vi "AuMT8852B SCO Input Sample Size.vi"(5 "Size (8-bit)":enum16{"8-bit", "16-bit"}(ring), 7 "Set/Get (Set)":enum16{"Set", "Get"}(ring), 8 "error in (no error)":errorcluster, 11 "VISA session":refnum<visa-resource-name>) -> (0 "error out":errorcluster, 2 "error code":i32, 3 "VISA session out":refnum<visa-resource-name>, 4 "Size out":enum16{"8-bit", "16-bit"}(ring))   [LabVIEW 2017]
doc: "Anritsu MT8852B Bluetooth Tester\n\nThis command is used to set the input sample size for the audio connection to either 8 bit or 16 bit. The value is only used by the MT885x when it is controlling an EUT via the front panel connection. The command can only be used when there is an ACL connection (and if the EUT is controlled via the front panel, no SCO connection).\n\nINPUTS\nSet/Get - whether the value is being sent to or retrieved from the instrument.\nSize - information to send to the instrument.\n\nOUTPUTS\nSize out - the present value in the instrument."
uses:
  <instrlib>/aumt8852B/General/Utilities/MT8850 Attribute ID.ctl
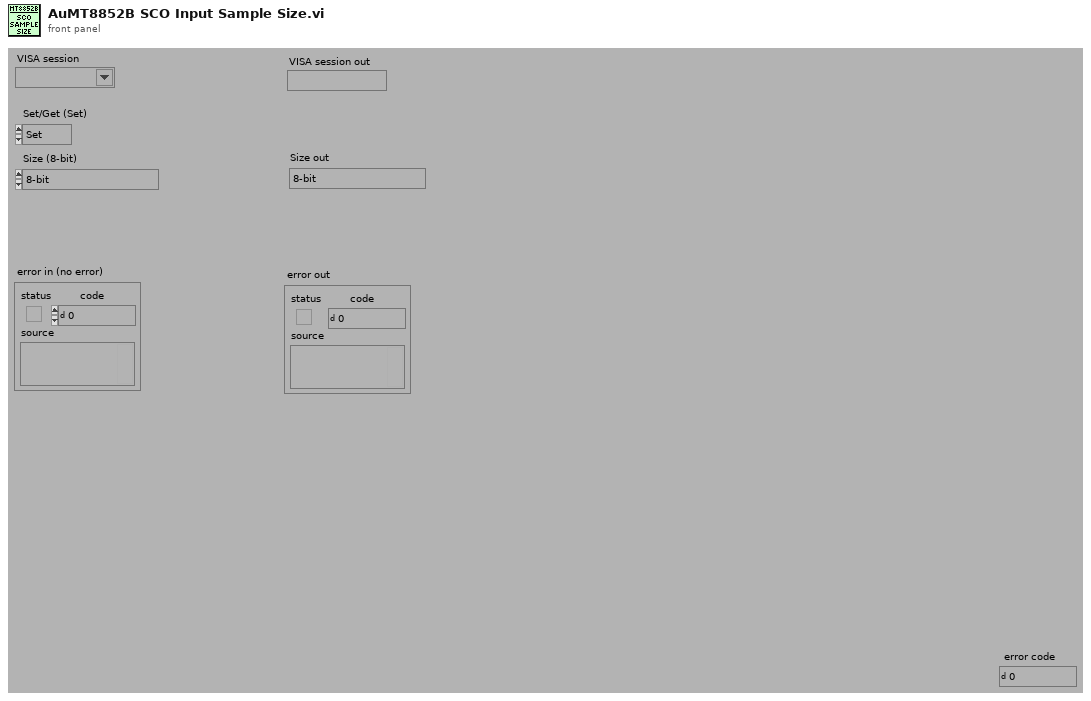
[diagram p1: front panel]
types:
  T1 = typedef "MT8850 Attribute ID.ctl" = enum16{"Operation mode", "Selected script", "EUT address source", "EUT Address", "EUT HCI RS232 Baud Rate", "Tester GPIB Address", "Tester RS232 Baud Rate", "Tester Bluetooth Address", "Tester Contrast", "Tester Key Click On", "Tester Modulation Index", "Tester Poll-Null Mode", "Tester Power Range", "Tester RS232 Mode", "Beep on Illegal Entry", "Display User Text", "User Text", "Calibration TX Modulation DAC", "Calibration RX Channel", "Calibration TX Channel", "Calibration TX Power", "Calibration Use TX Table", "Inquiry Request User-friendly Name", "Inquiry Number of Responses", "Inquiry Timeout", "Script Frequency Display", "Script Loop Count", "Script Loop Continuously", "Script Loop Stop on Fail", "Link timeout", "Page timeout", "Filter bandwidth", "SCO air code", "SCO bit position", "SCO input code", "SCO input data", "SCO input sample size", "SCO loopback mode", "SCO packet type", "SCO tone generator", "Tester page scan repetition mode", "Tester follow test mode", "Tester authentication state", "Tester authentication pin code", "Tester authentication pin length"}
  T2 = typedef "Attribute Status.ctl" = enum16{"No I/O needed", "I/O needed"}
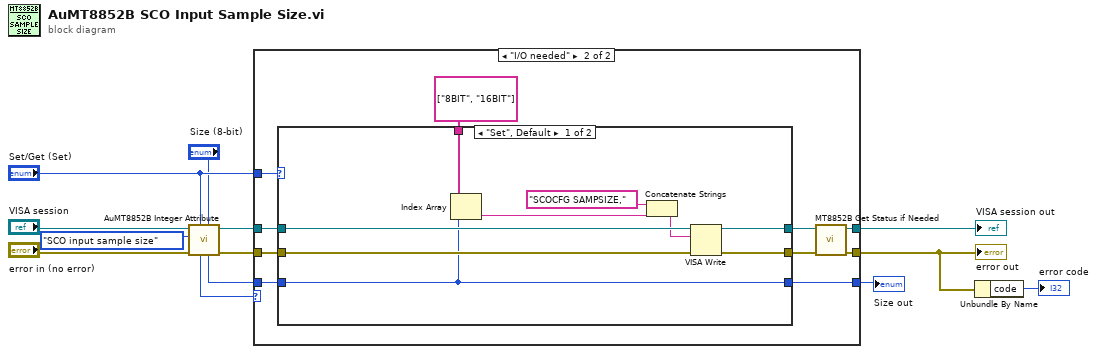
[diagram p0: block diagram]
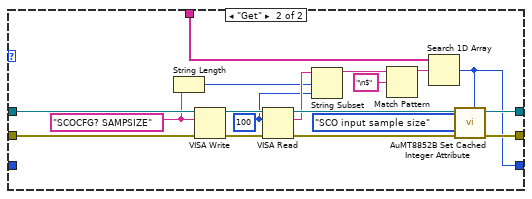
[diagram p3: hidden frame]
diagram:
  n1 = call <instrlib>:"AuMT8852B Integer Attribute.vi"("Value (0)"="Size (8-bit)", "Set/Get (Set)"="Set/Get (Set)", "error in (no error)"="error in (no error)", "Attribute ID"=MT8850_Attribute_ID."SCO input sample size", "VISA session"="VISA session") -> ("error out"=w6:errorcluster, "VISA session out"=w7:refnum<visa-resource-name>, "Value out"=w9:i32, "Status"=w4:T2)  [unwired: 3 in]
  n2 = case shown="\"I/O needed\"" w4 {
    tunnel: "Set/Get (Set)" -> [_ w25]
    tunnel: w9 -> [w16 w24]
    tunnel: [w14 w17] -> w1
    tunnel: [w15 w18] -> w8
    tunnel: w7 -> [w15 w23]
    tunnel: w6 -> [w14 w22]
    tunnel: [w16 w21] -> w3
    frame "No I/O needed", Default {
    }
    frame "I/O needed" {
      n3 = case shown="\"Set\", Default" w25 {
        tunnel: [w27 w45] -> w19
        tunnel: string[] ["8BIT", "16BIT"] ("Array Constant") -> [w35 w53]
        tunnel: w24 -> [w32 _]
        tunnel: [w28 w46] -> w20
        tunnel: w23 -> [w34 w52]
        tunnel: w22 -> [w33 w51]
        tunnel: [w32 w44] -> w21
        frame "Set", Default {
          n4 = Index Array(array=w35, index=w32) -> (element=w30:string)
          n5 = Concatenate Strings("SCOCFG SAMPSIZE," ("Substring"), w30) -> (w31:string)
          n6 = VISA Write(VISA resource name=w34, write buffer=w31, error in (no error)=w33) -> (VISA resource name out=w28:refnum<visa-resource-name>, error out=w27:errorcluster)  [unwired: 1 out]
        }
        frame "Get" {
          w36 = u32 100 ("byte count (0)")
          w42 = "SCOCFG? SAMPSIZE" ("write buffer (\"\")")
          n7 = String Length(string=w42) -> (length=w38:i32)
          n8 = VISA Write(VISA resource name=w52, write buffer=w42, error in (no error)=w51) -> (VISA resource name out=w50:refnum<visa-resource-name>, error out=w49:errorcluster)  [unwired: 1 out]
          n9 = VISA Read(VISA resource name=w50, byte count=w36, error in (no error)=w49) -> (VISA resource name out=w48:refnum<visa-resource-name>, read buffer=w39:string, error out=w47:errorcluster)  [unwired: 1 out]
          n10 = String Subset(string=w39, offset (0)=w38, length (rest)=w36) -> (substring=w37:string)
          n11 = Match Pattern(string=w37, regular expression="\n$") -> (before substring=w40:string)  [unwired: 1 in, 3 out]
          n12 = Search 1D Array(1D array=w53, element=w40) -> (index of element=w44:i32)  [unwired: 1 in]
          n13 = call <instrlib>:"AuMT8852B Set Cached Integer Attribute.vi"("Value (0)"=w44, "error in (no error)"=w47, "Attribute ID"=MT8850_Attribute_ID."SCO input sample size", "VISA session"=w48) -> ("error out"=w45:errorcluster, "VISA session out"=w46:refnum<visa-resource-name>)  [unwired: 6 in]
        }
      }
      n14 = call <instrlib>:"MT8852B Get Status if Needed.vi"("error in (no error)"=w19, "VISA session"=w20) -> ("error out"=w17:errorcluster, "VISA session out"=w18:refnum<visa-resource-name>)  [unwired: 8 in]
    }
  }
  "error out" <- w1
  "VISA session out" <- w8
  "Size out" <- w3
  n15 = Unbundle By Name(w1) -> ("code"=→"error code":i32)
